vi "Update.vi"(8 "error in (no error)":errorcluster, 11 "Timed Loop Controller in":refnum<class "Timed Loop Actor.lvclass">) -> (0 "error out":errorcluster, 3 "Timed Loop Controller out":refnum<class "Timed Loop Actor.lvclass">)   [LabVIEW 2025, in "Timed Loop Actor.lvlib" / "Timed Loop Actor.lvclass"]
doc: "This VI is a wrapper around Update Core.vi to provide the community scoped interface that the \"Update Msg.lvclass:Do.vi\" needs to invoke."
uses:
  Timed Loop Actor.lvclass
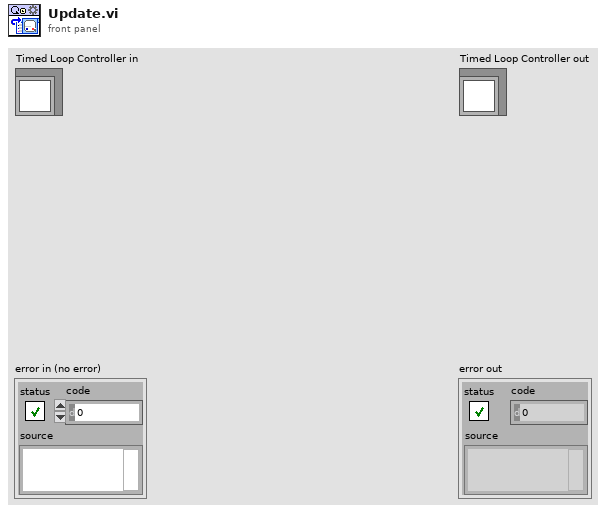
[diagram p1: front panel]
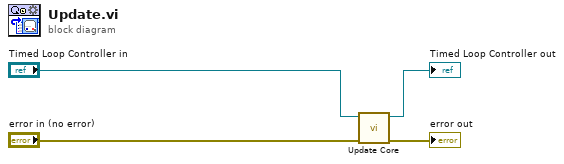
[diagram p0: block diagram]
diagram:
  n1 = call-dynamic "Update Core.vi"("error in (no error)"="error in (no error)", "Level Controller in"="Timed Loop Controller in") -> ("error out"=→"error out":errorcluster, "Level Controller out"=→"Timed Loop Controller out":refnum<class "Timed Loop Actor.lvclass">)  [unwired: 8 in]
